vi "Chart_to_GraphXY_3.vi"(7 "Function":T1, 8 "Error In":errorcluster, 10 "Time window":i32=100, 11 "Value In":T2) -> (0 "Error Out":errorcluster, 1 "XY Graph Speed":cluster{"Tempi":dbl[], "Valori":dbl[]}[](graph), 2 "XY Graph Current":cluster{"Tempi":dbl[], "Valori":dbl[]}[](graph), 3 "XY Graph Voltage":cluster{"Tempi":dbl[], "Valori":dbl[]}[](graph))   [LabVIEW 2015, in "My Graphs.lvlib"]
uses:
  My Graphs.lvlib
  Telemetria_Rotterdam_API_v2/TypeDef/data_graph.ctl
  Chart to Graph enum.ctl
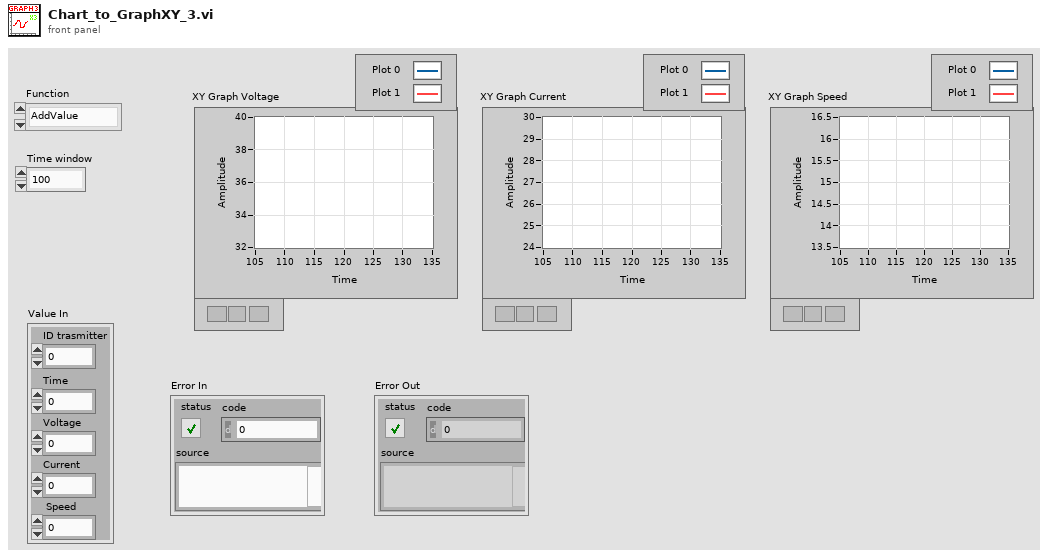
[diagram p1: front panel]
types:
  T1 = typedef "My Graphs.lvlib/Chart to Graph enum.ctl" = enum16{"AddValue", "Reset", "Delete_old"}
  T2 = typedef "data_graph.ctl" = cluster{"Time":sgl, "Voltage":sgl, "Current":sgl, " Speed":sgl, "ID trasmitter":u8}
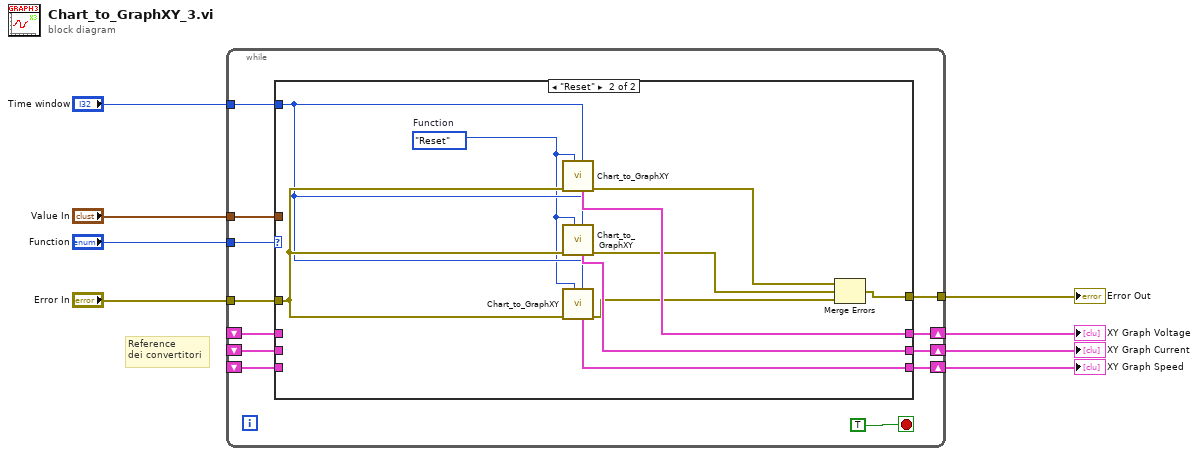
[diagram p0: block diagram]
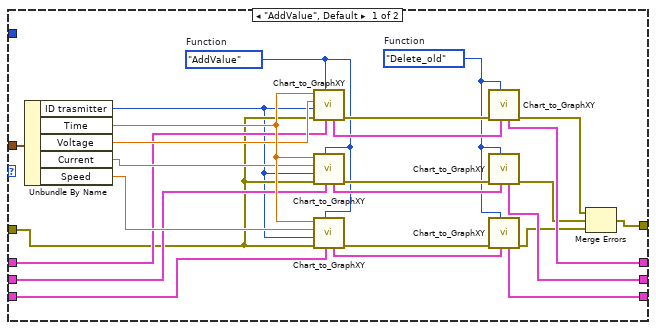
[diagram p2: hidden frame]
diagram:
  # "Reference\ndei convertitori"
  n1 = while {
    tunnel: "Error In" -> [w20]
    tunnel: [w19] -> w7
    tunnel: "Function" -> [w18]
    tunnel: "Value In" -> [w17]
    shift-right: [w10] -> w4
    shift-left: _ -> [w14]
    shift-right: [w11] -> w3
    shift-left: _ -> [w15]
    shift-right: [w12] -> w2
    shift-left: _ -> [w16]
    tunnel: "Time window" -> [w9]
    stop <- TRUE stop-if-true
    n2 = case shown="\"Reset\"" w18 {
      tunnel: w20 -> [w22 w51]
      tunnel: [w45 w55] -> w19
      tunnel: w17 -> [w44 _]
      tunnel: w16 -> [w23 _]
      tunnel: w15 -> [w37 _]
      tunnel: w14 -> [w38 _]
      tunnel: [w35 w54] -> w12
      tunnel: [w34 w53] -> w11
      tunnel: [w31 w52] -> w10
      tunnel: w9 -> [_ w47]
      frame "AddValue", Default {
        w24 = Chart_to_Graph_enum."AddValue"  # Function
        w25 = Chart_to_Graph_enum."Delete_old"  # Function
        n3 = Unbundle By Name(w44) -> ("ID trasmitter"=w21:u8, "Time"=w42:sgl, "Voltage"=w41:sgl, "Current"=w40:sgl, "Speed"=w39:sgl)
        n4 = call "Chart_to_GraphXY.vi"("reference in"=w38, "Function"=w24, "error in"=w22, "Index plot"=w21, "Valore in"=w41, "Tempo in"=w42) -> ("error out"=w43:errorcluster, "reference out"=w32:cluster{"Tempi":dbl[], "Valori":dbl[]}[])  [unwired: 1 in, 3 out]
        n5 = call "Chart_to_GraphXY.vi"("reference in"=w37, "Function"=w24, "error in"=w22, "Index plot"=w21, "Valore in"=w40, "Tempo in"=w42) -> ("error out"=w27:errorcluster, "reference out"=w33:cluster{"Tempi":dbl[], "Valori":dbl[]}[])  [unwired: 1 in, 3 out]
        n6 = call "Chart_to_GraphXY.vi"("reference in"=w23, "Function"=w24, "error in"=w22, "Index plot"=w21, "Valore in"=w39, "Tempo in"=w42) -> ("error out"=w26:errorcluster, "reference out"=w36:cluster{"Tempi":dbl[], "Valori":dbl[]}[])  [unwired: 1 in, 3 out]
        n7 = call "Chart_to_GraphXY.vi"("reference in"=w32, "Function"=w25, "error in"=w43) -> ("error out"=w30:errorcluster, "reference out"=w31:cluster{"Tempi":dbl[], "Valori":dbl[]}[])  [unwired: 4 in, 3 out]
        n8 = call "Chart_to_GraphXY.vi"("reference in"=w33, "Function"=w25, "error in"=w27) -> ("error out"=w29:errorcluster, "reference out"=w34:cluster{"Tempi":dbl[], "Valori":dbl[]}[])  [unwired: 4 in, 3 out]
        n9 = call "Chart_to_GraphXY.vi"("reference in"=w36, "Function"=w25, "error in"=w26) -> ("error out"=w28:errorcluster, "reference out"=w35:cluster{"Tempi":dbl[], "Valori":dbl[]}[])  [unwired: 4 in, 3 out]
        n10 = Merge Errors(w30, w29, w28) -> (w45:errorcluster)
      }
      frame "Reset" {
        w46 = Chart_to_Graph_enum."Reset"  # Function
        n11 = call "Chart_to_GraphXY.vi"("Time window"=w47, "Function"=w46, "error in"=w51) -> ("error out"=w50:errorcluster, "reference out"=w52:cluster{"Tempi":dbl[], "Valori":dbl[]}[])  [unwired: 4 in, 3 out]
        n12 = call "Chart_to_GraphXY.vi"("Time window"=w47, "Function"=w46, "error in"=w51) -> ("error out"=w49:errorcluster, "reference out"=w53:cluster{"Tempi":dbl[], "Valori":dbl[]}[])  [unwired: 4 in, 3 out]
        n13 = call "Chart_to_GraphXY.vi"("Time window"=w47, "Function"=w46, "error in"=w51) -> ("error out"=w48:errorcluster, "reference out"=w54:cluster{"Tempi":dbl[], "Valori":dbl[]}[])  [unwired: 4 in, 3 out]
        n14 = Merge Errors(w50, w49, w48) -> (w55:errorcluster)
      }
    }
  }
  "Error Out" <- w7
  "XY Graph Speed" <- w2
  "XY Graph Current" <- w3
  "XY Graph Voltage" <- w4
